vi "ACC Configuration Manager.vi"(0 "System Configuration In (Write, Update Only)":T2, 1 "Cfg File Path":path, 11 "Error In (no error)":errorcluster, 12 "Keys (Empty:All)":T1[](array[typedef]), 13 "Operation":T5) -> (4 "System Configuration Out":T2, 8 "Cancelled":bool, 15 "Error Out":errorcluster)   [LabVIEW 2011]
uses:
  Type Defs/ACTL Access Level Cluster.ctl
  Type Defs/ACTL Operator Cluster.ctl
  Type Defs/ACTL Access Level Enum.ctl
  Type Defs/ACTL Configuration Operation Enum.ctl
  Type Defs/ACTL Configuration Enum.ctl
  Configuration Files/Type Defs/CFG File Operation Enum.ctl
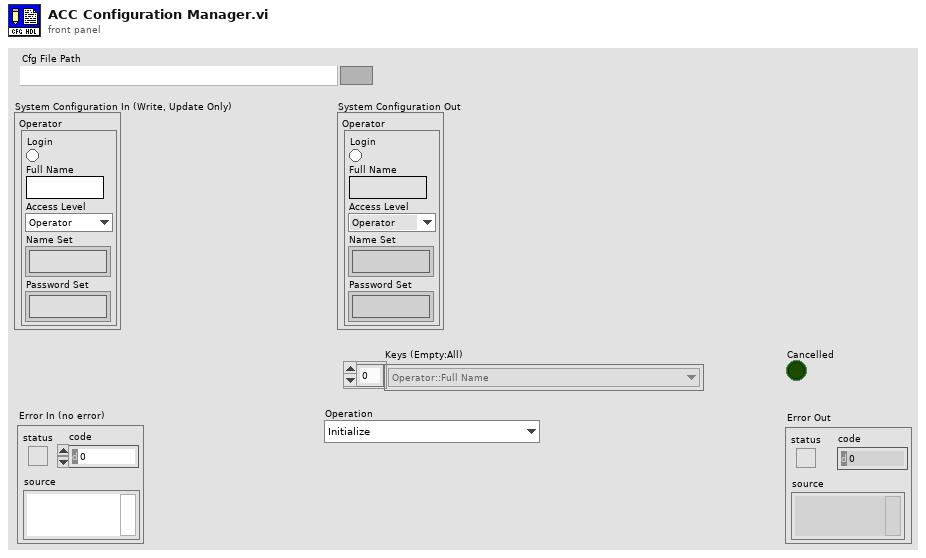
[diagram p1: front panel]
types:
  T1 = typedef "ACTL Configuration Enum.ctl" = enum16{"Operator::Full Name", "Operator::Login", "Operator::Access Level", "Operator::Name Set", "Operator::Password Set"}
  T2 = typedef "ACTL Access Level Cluster.ctl" = cluster{"Operator":T3}
  T3 = typedef "ACTL Operator Cluster.ctl" = cluster{"Full Name":string, "Access Level":T4, "Name Set":string[], "Login":bool, "Password Set":string[]}
  T4 = typedef "ACTL Access Level Enum.ctl" = enum16{"Operator", "Technician", "Engineer", "Programmer"}
  T5 = typedef "ACTL Configuration Operation Enum.ctl" = enum16{"Initialize", "Get Status", "Read", "Write", "Update", "Copy", "Edit"}
  T6 = typedef "CFG File Operation Enum.ctl" = enum16{"Read", "Write", "Copy", "Edit"}
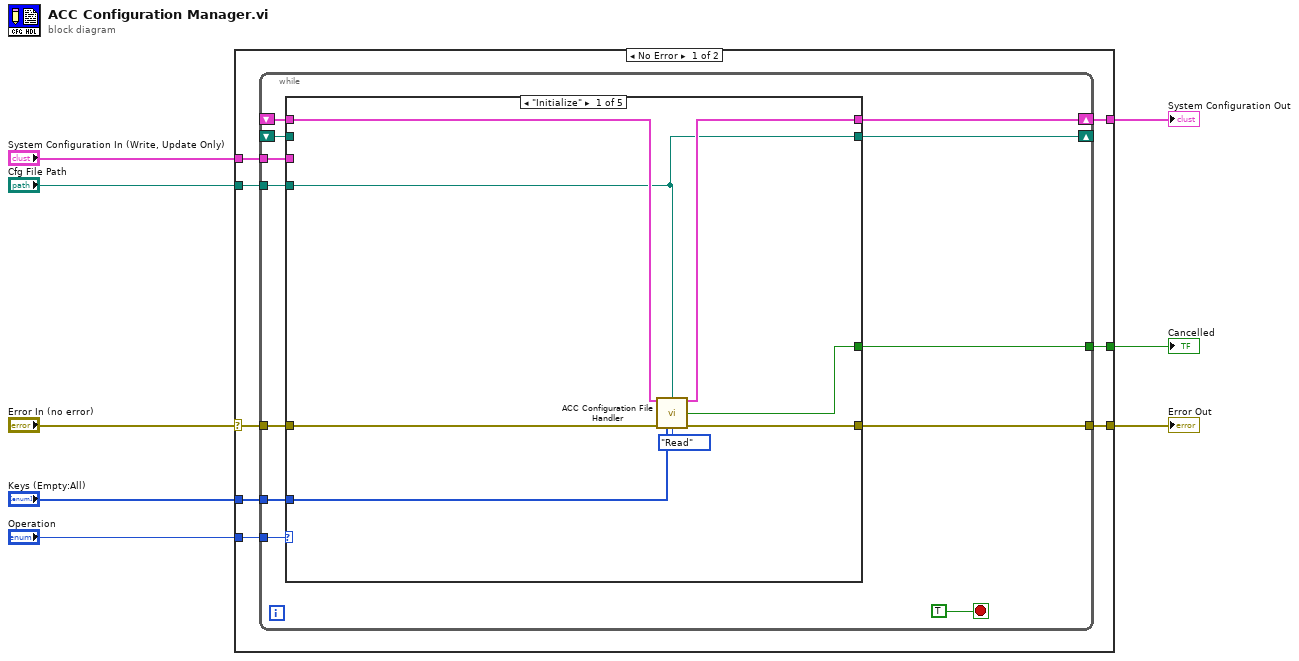
[diagram p0: block diagram]
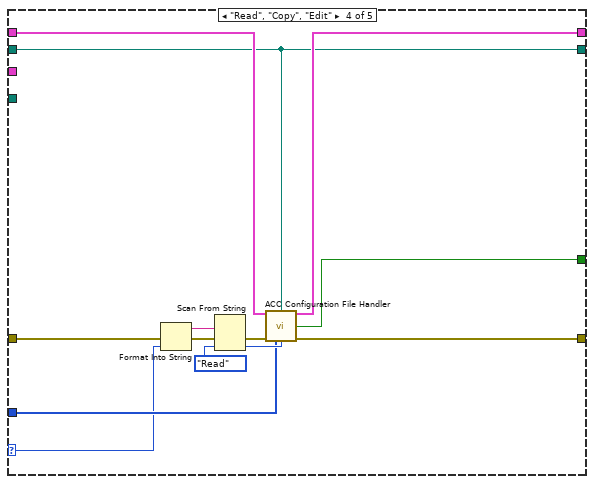
[diagram p4: hidden frame]
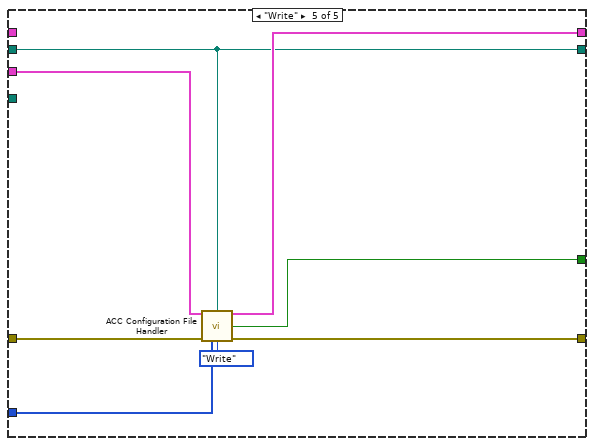
[diagram p5: hidden frame]
diagram:
  n1 = case shown="No Error" "Error In (no error)" {
    selector: "Error In (no error)" -> [w16 w65]
    tunnel: [w15 w65] -> w3
    tunnel: "Operation" -> [w13 _]
    tunnel: [w12 w64] -> w2
    tunnel: "System Configuration In (Write, Update Only)" -> [w10 w64]
    tunnel: "Keys (Empty:All)" -> [w11 _]
    tunnel: [w14 _] -> w4
    tunnel: "Cfg File Path" -> [w9 _]
    frame No Error {
      n2 = while {
        tunnel: w16 -> [w27]
        tunnel: [w20] -> w15
        tunnel: [w28] -> w14
        shift-right: [w21] -> w12
        shift-left: _ -> [w23]
        tunnel: w13 -> [w25]
        tunnel: w10 -> [w24]
        tunnel: w11 -> [w22]
        tunnel: w9 -> [w19]
        shift-right: [w18] -> _
        shift-left: _ -> [w17]
        stop <- TRUE stop-if-true
        n3 = case shown="\"Initialize\"" w25 {
          selector: w25 -> [_ _ _ w47 _]
          tunnel: [w33 w38 w42 w45 w57] -> w20
          tunnel: [w35 _ _ w46 w63] -> w28
          tunnel: [w30 w39 w41 w44 w58] -> w21
          tunnel: w27 -> [w32 w38 w42 w52 w61]
          tunnel: w24 -> [_ _ w41 _ w59]
          tunnel: w23 -> [w31 w39 _ w48 _]
          tunnel: w22 -> [w34 _ _ w49 w62]
          tunnel: w19 -> [w29 _ _ _ _]
          tunnel: [w29 w37 w40 w43 w56] -> w18
          tunnel: w17 -> [_ w37 w40 w43 w56]
          frame "Initialize" {
            n4 = call "ACC Configuration File Handler.vi"("Operator"=w31, "Cfg File Path"=w29, "Error In (no error)"=w32, "Keys (Empty:All)"=w34, "Operation"=CFG_File_Operation_Enum."Read") -> ("System Configuration Out"=w30:T2, "Cancelled"=w35:bool, "Error Out"=w33:errorcluster)  [unwired: 2 in, 6 out]
          }
          frame "Get Status" {
          }
          frame "Update" {
          }
          frame "Read", "Copy", "Edit" {
            n5 = Format Into String(error in=w52, w47) -> (resulting string=w55:string, error out=w51:errorcluster)  [unwired: 2 in]
            n6 = Scan From String(input string=w55, error in=w51, default 1=CFG_File_Operation_Enum."Read" ("Operation")) -> (error out=w50:errorcluster, output 1=w53:T6)  [unwired: 2 in, 2 out]
            n7 = call "ACC Configuration File Handler.vi"("Operator"=w48, "Cfg File Path"=w43, "Error In (no error)"=w50, "Keys (Empty:All)"=w49, "Operation"=w53) -> ("System Configuration Out"=w44:T2, "Cancelled"=w46:bool, "Error Out"=w45:errorcluster)  [unwired: 2 in, 6 out]
          }
          frame "Write" {
            n8 = call "ACC Configuration File Handler.vi"("Operator"=w59, "Cfg File Path"=w56, "Error In (no error)"=w61, "Keys (Empty:All)"=w62, "Operation"=CFG_File_Operation_Enum."Write") -> ("System Configuration Out"=w58:T2, "Cancelled"=w63:bool, "Error Out"=w57:errorcluster)  [unwired: 2 in, 6 out]
          }
        }
      }
    }
    frame Error {
    }
  }
  "System Configuration Out" <- w2
  "Error Out" <- w3
  "Cancelled" <- w4
